vi "Write Configuration.vi"(3 "Configuration":T1={"DAQmxChannel myVolt"={"DAQmxChannel myVinput1"={"PhysicalChanName"="", "AI_Voltage_Units"=10348, "AI_Max"=5.0, "AI_Min"=-5.0}, "DAQmxChannel myVinput2"={"PhysicalChanName"="", "AI_Voltage_Units"=10348, "AI_Max"=5.0, "AI_Min"=-5.0}, "DAQmxChannel myVoutput1"={"PhysicalChanName"="", "AI_Min"=-5.0, "AI_Max"=5.0, "AI_Voltage_Units"=10348}, "DAQmxChannel myVoutput2"={"PhysicalChanName"="", "AI_Min"=-5.0, "AI_Max"=5.0, "AI_Voltage_Units"=10348}, "Saidmple Clock Input"={"rate"=1000.0, "samples per channel"=100}, "Saidmple Clock Output"={"rate"=1000.0, "samples per channel"=100}}, "Dev"=""} {"DAQmxChannel myVolt"."DAQmxChannel myVoutput2"."AI_Voltage_Units" items=["伏特"=10348, "来自自定义换算"=10065]; "DAQmxChannel myVolt"."DAQmxChannel myVoutput1"."AI_Voltage_Units" items=["伏特"=10348, "来自自定义换算"=10065]; "DAQmxChannel myVolt"."DAQmxChannel myVinput1"."AI_Voltage_Units" items=["伏特"=10348, "来自自定义换算"=10065]; "DAQmxChannel myVolt"."DAQmxChannel myVinput2"."AI_Voltage_Units" items=["伏特"=10348, "来自自定义换算"=10065]}, 8 "error in (no error)":errorcluster, 11 "文件名":string="jd-solution-1.xml") -> (0 "error out":errorcluster)   [LabVIEW 2016]
uses:
  Contral/Coniguration.ctl
  <vilib>/NI/GXML/GXML.lvlib
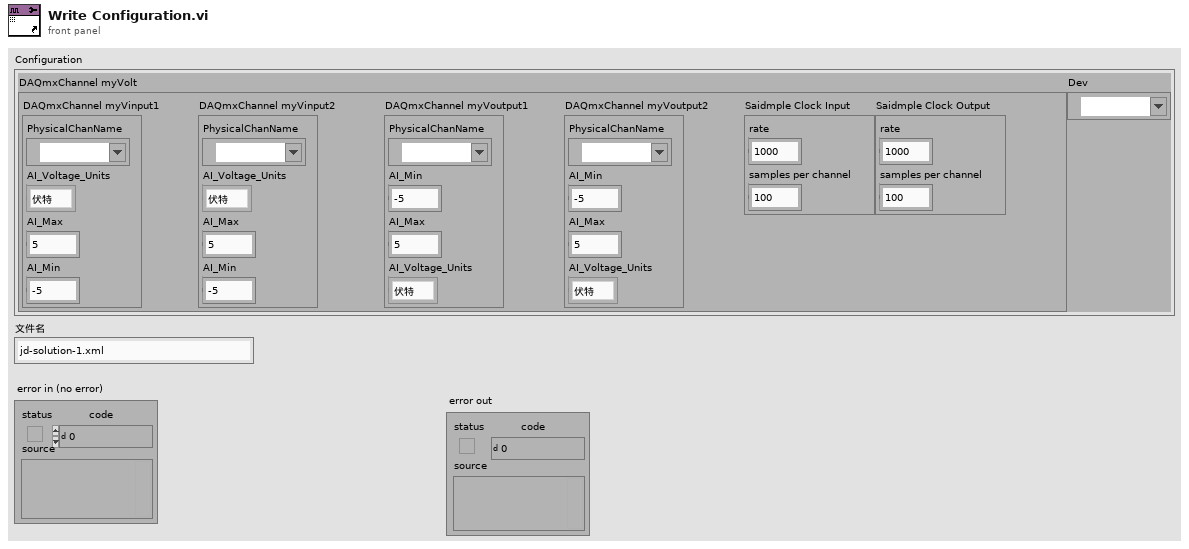
[diagram p1: front panel]
types:
  T1 = typedef "Coniguration.ctl" = cluster{"DAQmxChannel myVolt":cluster{"DAQmxChannel myVinput1":cluster{"PhysicalChanName":tag, "AI_Voltage_Units":i32, "AI_Max":dbl, "AI_Min":dbl}, "DAQmxChannel myVinput2":cluster{"PhysicalChanName":tag, "AI_Voltage_Units":i32, "AI_Max":dbl, "AI_Min":dbl}, "DAQmxChannel myVoutput1":cluster{"PhysicalChanName":tag, "AI_Min":dbl, "AI_Max":dbl, "AI_Voltage_Units":i32}, "DAQmxChannel myVoutput2":cluster{"PhysicalChanName":tag, "AI_Min":dbl, "AI_Max":dbl, "AI_Voltage_Units":i32}, "Saidmple Clock Input":cluster{"rate":dbl, "samples per channel":i32}, "Saidmple Clock Output":cluster{"rate":dbl, "samples per channel":i32}}, "Dev":tag}
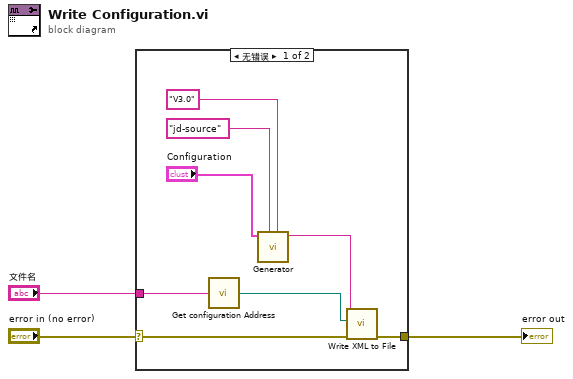
[diagram p0: block diagram]
diagram:
  n1 = case shown="无错误" "error in (no error)" {
    selector: "error in (no error)" -> [w4 w12]
    tunnel: "文件名" -> [w11 _]
    tunnel: [w6 w12] -> w2
    frame No Error {
      n2 = call "Get configuration Address.vi"("文件名"=w11) -> ("配置文件路径"=w5:path)
      n3 = call <vilib>:"Generator.vi"("Version String"="V3.0", "Version Tag Name"="jd-source", "Variant"="Configuration") -> ("XML String Out"=w7:string)  [unwired: 7 in, 1 out]
      n4 = call <vilib>:"Write XML to File.vi"("error in"=w4, "XML File Path"=w5, "XML Input"=w7) -> ("error out"=w6:errorcluster)  [unwired: 8 in]
    }
    frame Error {
    }
  }
  "error out" <- w2
